vi "Calculate.vi"(5 "WFGraph Refnum":refnum<vi>, 7 "Measurement info":T2={"Det index"=0, "Clk index"=1, "Avg range"=1e-08}, 8 "error in":errorcluster, 9 "Changed reg":u8, 10 "Polarity":T1, 11 "file (use dialog)":path) -> (0 "error out":errorcluster, 2 "Settling time 5% (us)":dbl, 3 "Transition duration 10% (us)":dbl, 4 "Waveform data out":cluster{"t0":dbl, "dt":dbl, "Y":dbl[]}[](graph), 6 "Timing measurements":T3 {"measurement info 10%"."ref levels"."ref units" items=["absolute", "relative"]; "measurement info 5%"."ref levels"."ref units" items=["absolute", "relative"]})   [LabVIEW 2020]
uses:
  Timing measurements.ctl
  <vilib>/Waveform/WDTOps.llb/WDT Get Waveform Time Array DBL.vi
  <vilib>/measure/mascope.llb/Amplitude and Levels 1 chan.vi
  <vilib>/measure/mascope.llb/Transition Measurements 1 chan.vi
  <vilib>/Waveform/WDTOps.llb/WDT Waveform Duration DBL.vi
  <vilib>/Waveform/WDTOps.llb/WDT Get Waveform Subset DBL.vi
  <vilib>/Waveform/DWDTOps.llb/DWDT Analog to Digital.vi
  <vilib>/Waveform/DWDTOps.llb/DWDT Digital to Boolean Array.vi
  <vilib>/measure/NI_MAPro.lvlib
panel:
  out "full-scale range (pk-pk)":dbl=1.8
  out "# of clk edge":i32
  out "t0 to 10% (us)":dbl
  out "t0 to 5% (us)":dbl
  out "Settling index":i32
  out "measurement info 5%":T4 {"ref levels"."ref units" items=["absolute", "relative"]; "ref levels"."high ref level" format="%.2p"; "ref levels"."low ref level" format="%.2p"; "ref levels"."mid ref level" format="%.2p"; "end time" format="%.2p"; "start time" format="%.2p"}
  out "post-transition 5%":T5
  out "pre-transition 5%":T5
  out "slope 5%":dbl
  out "transition duration 5%":dbl
  out "amplitude":dbl format="%.2p"
  out "high state level":dbl format="%.2g"
  out "low state level":dbl format="%.2g"
  out "slope 10%":dbl
  out "measurement info 10%":T4 {"ref levels"."ref units" items=["absolute", "relative"]; "ref levels"."high ref level" format="%.2p"; "ref levels"."low ref level" format="%.2p"; "ref levels"."mid ref level" format="%.2p"; "end time" format="%.2p"; "start time" format="%.2p"}
  out "pre-transition 10%":T5
  out "Post-transition 10%":T5
  out "t0 (s)":dbl
  out "Digital Waveform Graph":digitalwaveform(graph)
  out "t0 index":i32
  # "Standard frame: 22nd\nExtended frame: 31st and 40th"
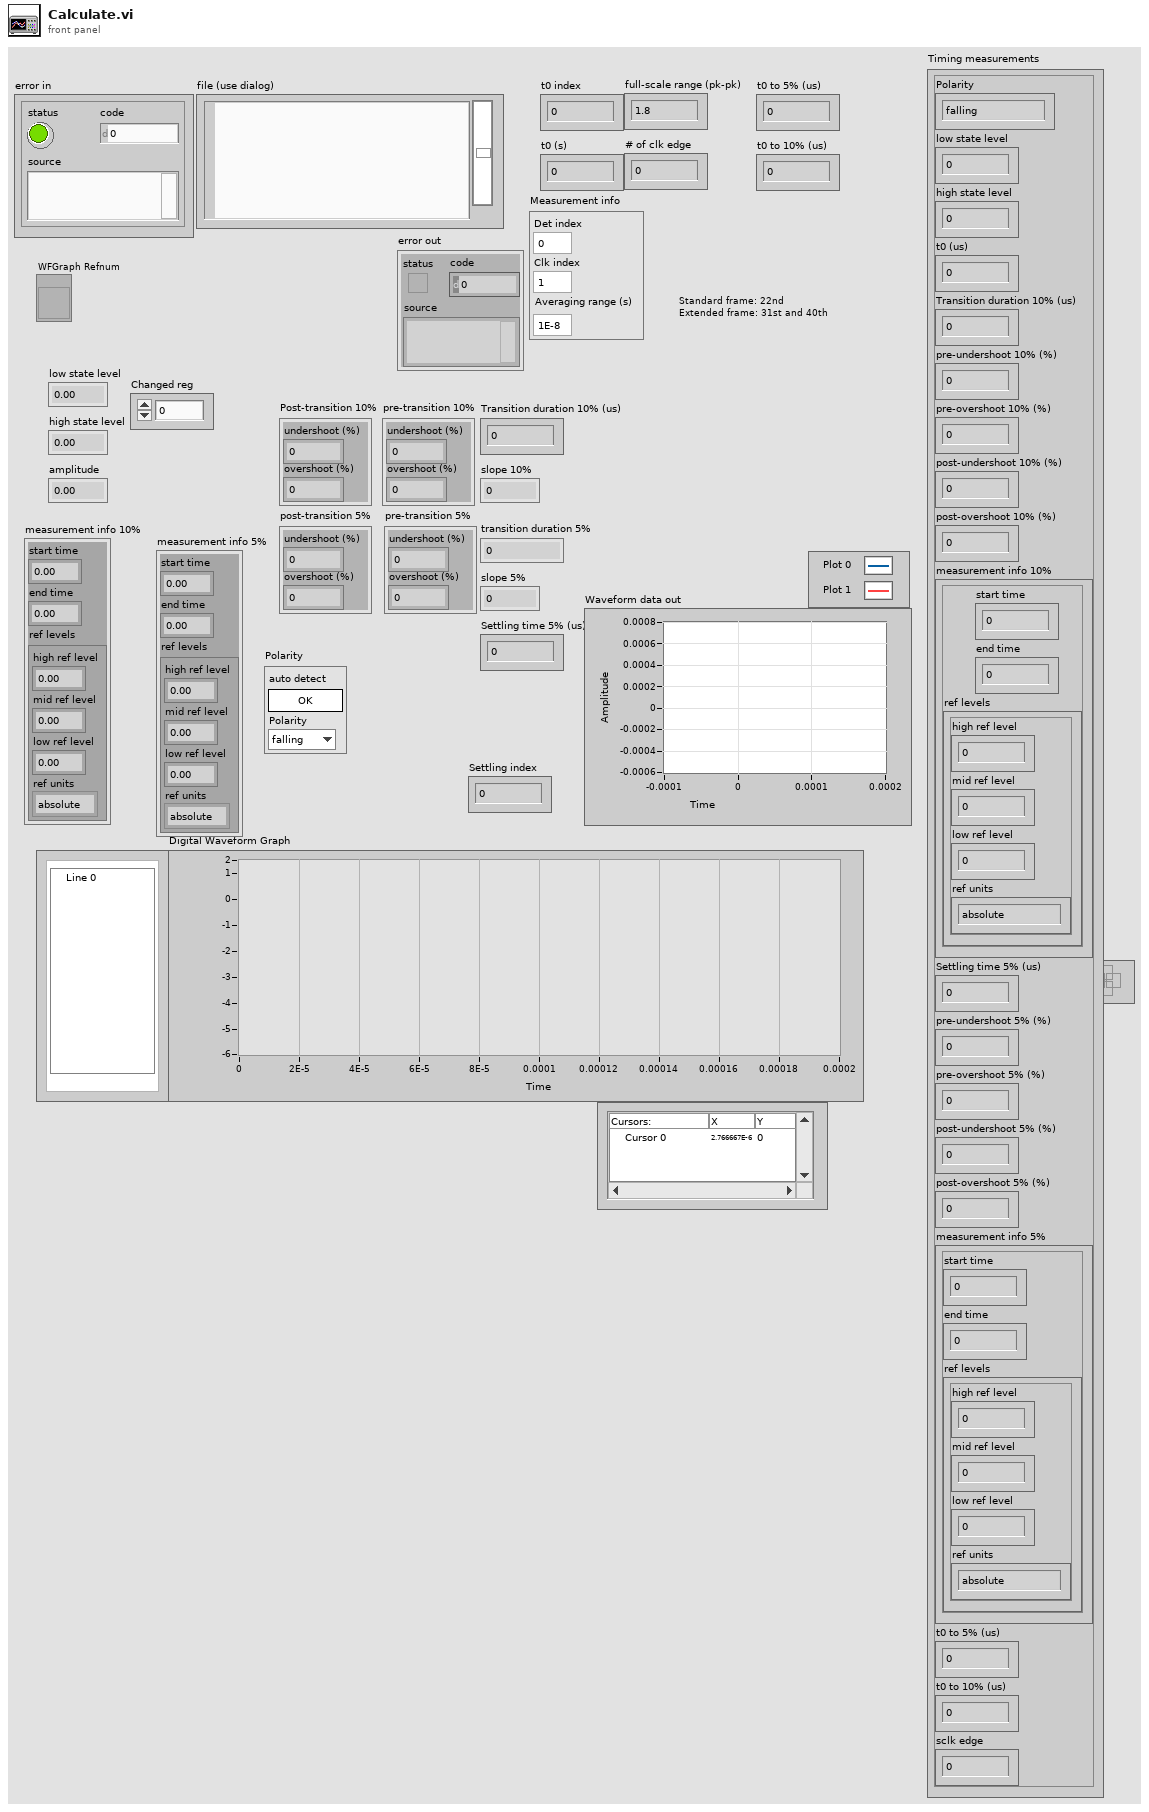
[diagram p1: front panel]
types:
  T1 = cluster{"auto detect":bool, "Polarity":enum16{"falling", "rising"}}
  T2 = cluster{"Det index":i32, "Clk index":i32, "Avg range":dbl}
  T3 = typedef "Timing measurements.ctl" = cluster{"Polarity":enum16{"falling", "rising"}, "low state level":dbl, "high state level":dbl, "t0 (us)":dbl, "Transition duration 10% (us)":dbl, "pre-undershoot 10% (%)":dbl, "pre-overshoot 10% (%)":dbl, "post-undershoot 10% (%)":dbl, "post-overshoot 10% (%)":dbl, "measurement info 10%":cluster{"start time":dbl, "end time":dbl, "ref levels":cluster{"high ref level":dbl, "mid ref level":dbl, "low ref level":dbl, "ref units":u16}}, "Settling time 5% (us)":dbl, "pre-undershoot 5% (%)":dbl, "pre-overshoot 5% (%)":dbl, "post-undershoot 5% (%)":dbl, "post-overshoot 5% (%)":dbl, "measurement info 5%":cluster{"start time":dbl, "end time":dbl, "ref levels":cluster{"high ref level":dbl, "mid ref level":dbl, "low ref level":dbl, "ref units":u16}}, "t0 to 5% (us)":dbl, "t0 to 10% (us)":dbl, "sclk edge":i32}
  T4 = cluster{"start time":dbl, "end time":dbl, "ref levels":cluster{"high ref level":dbl, "mid ref level":dbl, "low ref level":dbl, "ref units":u16}}
  T5 = cluster{"undershoot (%)":dbl, "overshoot (%)":dbl}
  T6 = cluster{"method":enum32{"histogram", "peak", "auto select"}, "histogram size":i32, "histogram method":enum16{"mode"}, "reserved":dbl}
  T7 = cluster{"high ref level":dbl, "mid ref level":dbl, "low ref level":dbl, "ref units":u16}
  T8 = typedef "imagedata.ctl" = cluster{"image type":i32, "image depth":i32, "image":u8[], "mask":u8[], "colors":u32[], "Rectangle":cluster{"left":i16, "top":i16, "right":i16, "bottom":i16}}
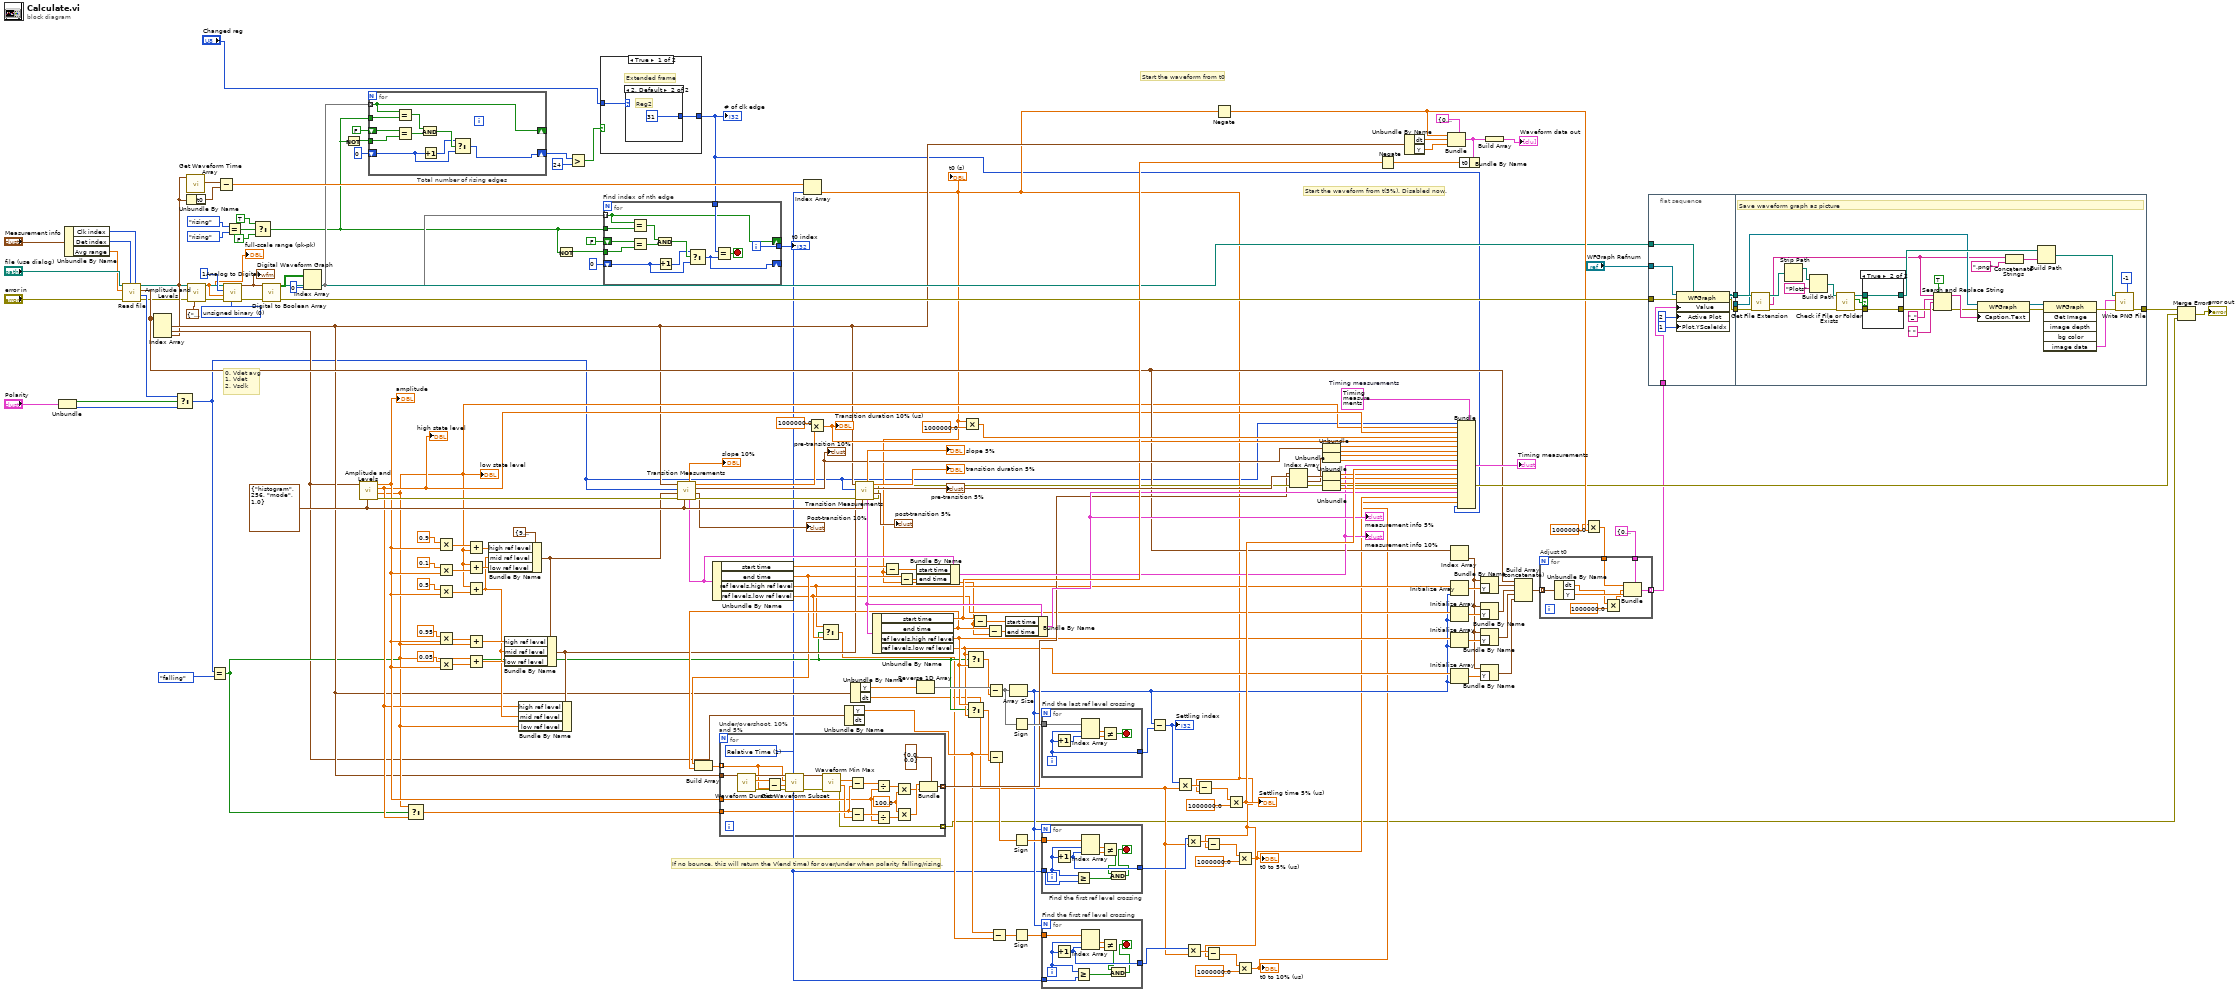
[diagram p0: block diagram]
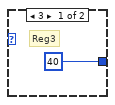
[diagram p2: hidden frame]
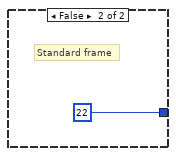
[diagram p3: hidden frame]
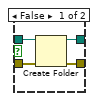
[diagram p4: hidden frame]
diagram:
  w117 = T3 {"Polarity"=enum."rising", "low state level"=0.0, "high state level"=0.0, "t0 (us)"=0.0, "Transition duration 10% (us)"=0.0, "pre-undershoot 10% (%)"=0.0, "pre-overshoot 10% (%)"=0.0, "post-undershoot 10% (%)"=0.0, "post-overshoot 10% (%)"=0.0, "measurement info 10%"={"start time"=0.0, "end time"=0.0, "ref levels"={"high ref level"=0.0, "mid ref level"=0.0, "low ref level"=0.0, "ref units"=0}}, "Settling time 5% (us)"=0.0, "pre-undershoot 5% (%)"=0.0, "pre-overshoot 5% (%)"=0.0, "post-undershoot 5% (%)"=0.0, "post-overshoot 5% (%)"=0.0, "measurement info 5%"={"start time"=0.0, "end time"=0.0, "ref levels"={"high ref level"=0.0, "mid ref level"=0.0, "low ref level"=0.0, "ref units"=0}}, "t0 to 5% (us)"=0.0, "t0 to 10% (us)"=0.0, "sclk edge"=0}  # Timing measurements
  w140 = T6 {"method"=enum."histogram", "histogram size"=256, "histogram method"=enum."mode", "reserved"=1.0} ("state settings")
  w177 = u16 0 items=["unsigned binary", "offset binary", "2's complement"] ("data format (offset binary)")
  # "If no bounce, this will return the V(end time) for over/under when polarity falling/rising."
  # "0. Vdet avg\n1. Vdet\n2. Vsclk"
  # "Start the waveform from t(5%). Disabled now."
  # "Start the waveform from t0"
  n1 = Unbundle("Polarity") -> ("auto detect"=w21:bool, "Polarity"=w20:enum16{"falling", "rising"})
  n2 = Unbundle By Name("Measurement info") -> ("Clk index"=w28:i32, "Det index"=w27:i32, "Avg range"=w2:dbl)
  n3 = call "Read file.vi"("Clk index"=w28, "Det index"=w27, "error in (no error)"="error in", "Averaging range"=w2, "file (use dialog) in"="file (use dialog)") -> ("Error Out"=w3:errorcluster, "Polarity"=w19:enum16{"falling", "rising"}, "Waveform Array"=w68:waveform(dbl)[], "file (use dialog) out"=w69:path)  [unwired: 3 in]
  n4 = Index Array(array=w68) -> (element #1=w58:waveform(dbl), element #2=w33:waveform(dbl), element #3=w7:waveform(dbl))  [unwired: 3 in]
  n5 = Select(t=w19, s=w21, f=w20) -> (s? t:f=w18:enum16{"falling", "rising"})
  n6 = call-poly <vilib>:"Get Waveform Time Array.vi"("waveform in"=w7) -> ("X array"=w170:timestamp[])  [unwired: 9 in, 1 out]
  n7 = Unbundle By Name(w7) -> ("t0"=w171:timestamp)
  n8 = call-poly <vilib>:"Amplitude and Levels.vi"("state settings"=T6 {"method"=enum."histogram", "histogram size"=256, "histogram method"=enum."mode", "reserved"=1.0}, "error in (no error)"=w3, "signal in"=w7) -> ("error out"=w6:errorcluster, "amplitude"=w4:dbl)  [unwired: 5 in, 2 out]
  "full-scale range (pk-pk)" <- w4
  n9 = Equal?(x=w18, y=enum16{"falling", "rising"}."falling" ("Polarity 2")) -> (x = y?=w45:bool)
  n10 = Subtract(x=w170, y=w171) -> (x-y=w169:dbl[])
  n11 = call-poly <vilib>:"Analog to Digital.vi"("data format (offset binary)"=w177, "error in (no error)"=w6, "full-scale range (pk-pk)"=w4, "resolution (16 bit)"=1, "analog waveform"=w7) -> ("error out"=w176:errorcluster, "digital waveform"=w152:digitalwaveform)  [unwired: 3 in, 2 out]
  "Digital Waveform Graph" <- w152
  n12 = Equal?(x=enum16{"falling", "rising"}."rising" ("clk edge"), y=enum16{"falling", "rising"}."rising") -> (x = y?=w136:bool)
  n13 = Select(t=TRUE ("x"), s=w136, f=FALSE ("y")) -> (s? t:f=w12:bool)
  n14 = call-poly <vilib>:"Digital to Boolean Array.vi"("error in (no error)"=w176, "digital waveform"=w152) -> ("error out"=w159:errorcluster, "boolean array"=w173:bool[][])  [unwired: 8 in]
  n15 = Index Array(array=w173, index (col)=0 ("disabled index (col)")) -> (element=w14:bool[])  [unwired: 1 in]
  n16 = Not(x=w12) -> (.not. x?=w13:bool)
  n17 = call-poly <vilib>:"Amplitude and Levels.vi"("state settings"=w140, "signal in"=w33) -> ("error out"=w162:errorcluster, "low state level"=w63:dbl, "high state level"=w65:dbl, "amplitude"=w78:dbl)  [unwired: 6 in]
  "low state level" <- w63
  "high state level" <- w65
  "amplitude" <- w78
  n18 = for "Total number of rising edges" {
    shift-right: [w181] -> _
    shift-left: FALSE ("Boolean") -> [w182]
    tunnel: w14 -> [w181] mode=indexing
    shift-right: [w184] -> w9
    shift-left: 0 -> [w185]
    tunnel: w12 -> [w180]
    tunnel: w13 -> [w179]
    n19 = Equal?(x=w181, y=w180) -> (x = y?=w188:bool)
    n20 = Equal?(x=w182, y=w179) -> (x = y?=w183:bool)
    n21 = And(x=w188, y=w183) -> (x .and. y?=w187:bool)
    n22 = Increment(x=w185) -> (x+1=w186:i32)
    n23 = Select(t=w186, s=w187, f=w185) -> (s? t:f=w184:i32)
  }
  n24 = Select(t=w63, s=w45, f=w65) -> (s? t:f=w79:dbl)
  n25 = Multiply(x=0.9, y=w78) -> (x*y=w93:dbl)
  n26 = Multiply(x=0.1, y=w78) -> (x*y=w94:dbl)
  n27 = Multiply(x=0.5, y=w78) -> (x*y=w85:dbl)
  n28 = Multiply(x=0.95, y=w78) -> (x*y=w92:dbl)
  n29 = Multiply(x=0.05, y=w78) -> (x*y=w91:dbl)
  n30 = Add(x=w93, y=w63) -> (x+y=w87:dbl)
  n31 = Add(x=w63, y=w94) -> (x+y=w88:dbl)
  n32 = Add(x=w63, y=w85) -> (x+y=w66:dbl)
  n33 = Add(x=w92, y=w63) -> (x+y=w89:dbl)
  n34 = Add(x=w63, y=w91) -> (x+y=w90:dbl)
  n35 = Bundle By Name(cluster=T7 {"high ref level"=90.0, "mid ref level"=50.0, "low ref level"=10.0, "ref units"=0} ("reference levels"), "high ref level"=w87, "mid ref level"=w66, "low ref level"=w88) -> (w84:T7)
  n36 = Bundle By Name(cluster=w84, "high ref level"=w89, "mid ref level"=w66, "low ref level"=w90) -> (w64:T7)
  n37 = Bundle By Name(cluster=w64, "high ref level"=w65, "mid ref level"=w66, "low ref level"=w63) -> ()  [unwired: 1 out]
  n38 = Not(x=w12) -> (.not. x?=w135:bool)
  n39 = Greater?(x=w9, y=24) -> (0:w10:bool)
  n40 = case shown="True" w10 {
    tunnel: [w190 22 ("# of clk edge")] -> w8
    tunnel: "Changed reg" -> [w189 _]
    frame True {
      # "Extended frame"
      n41 = case shown="2, Default" w189 {
        tunnel: [40 ("# of clk edge") 31 ("# of clk edge")] -> w190
        frame 3 {
          # "Reg3"
        }
        frame 2, Default {
          # "Reg2"
        }
      }
    }
    frame False {
      # "Standard frame"
    }
  }
  "# of clk edge" <- w8
  n42 = for "Find index of nth edge" {
    shift-right: [w197] -> _
    shift-left: FALSE ("Boolean") -> [w198]
    tunnel: w14 -> [w197] mode=indexing
    shift-right: [w201] -> _
    shift-left: 0 -> [w203]
    tunnel: w8 -> [w200]
    tunnel: [w196] -> w30
    tunnel: w12 -> [w195]
    tunnel: w135 -> [w194]
    i -> [w196]
    stop <- w202 stop-if-true
    n43 = Equal?(x=w197, y=w195) -> (x = y?=w206:bool)
    n44 = Equal?(x=w198, y=w194) -> (x = y?=w199:bool)
    n45 = And(x=w206, y=w199) -> (x .and. y?=w205:bool)
    n46 = Increment(x=w203) -> (x+1=w204:i32)
    n47 = Select(t=w204, s=w205, f=w203) -> (s? t:f=w201:i32)
    n48 = Equal?(x=w200, y=w201) -> (x = y?=w202:bool)
  }
  "t0 index" <- w30
  n49 = call-poly <vilib>:"Transition Measurements.vi"("percent level settings"=w140, "error in (no error)"=w162, "reference levels"=w84, "polarity (rising)"=w18, "signal in"=w58) -> ("error out"=w100:errorcluster, "post-transition"=→"Post-transition 10%":T5, "pre-transition"=w124:T5, "transition duration"=w163:dbl, "measurement info"=w110:T4, "slope"=→"slope 10%":dbl)  [unwired: 1 in]
  "pre-transition 10%" <- w124
  n50 = Unbundle By Name(w110) -> ("start time"=w80:dbl, "end time"=w62:dbl, "ref levels.high ref level"=w46:dbl, "ref levels.low ref level"=w47:dbl)
  n51 = Index Array(array=w169, index=w30) -> (element=w34:dbl)
  "t0 (s)" <- w34
  n52 = Multiply(x=1000000.0 ("y"), y=w163) -> (x*y=w101:dbl)
  "Transition duration 10% (us)" <- w101
  n53 = Select(t=w46, s=w45, f=w47) -> (s? t:f=w43:dbl)
  n54 = Unbundle By Name(w33) -> ("Y"=w44:dbl[])  [unwired: 1 out]
  n55 = Unbundle By Name(w58) -> ("Y"=w48:dbl[], "dt"=w35:dbl)
  n56 = call-poly <vilib>:"Transition Measurements.vi"("percent level settings"=w140, "error in (no error)"=w100, "reference levels"=w64, "polarity (rising)"=w18, "signal in"=w58) -> ("error out"=w81:errorcluster, "post-transition"=→"post-transition 5%":T5, "pre-transition"=w123:T5, "transition duration"=→"transition duration 5%":dbl, "measurement info"=w105:T4, "slope"=→"slope 5%":dbl)  [unwired: 1 in]
  "pre-transition 5%" <- w123
  n57 = Unbundle By Name(w105) -> ("start time"=w104:dbl, "end time"=w77:dbl, "ref levels.high ref level"=w57:dbl, "ref levels.low ref level"=w56:dbl)
  n58 = Build Array(w62, w77) -> (w76:dbl[])
  n59 = for "Under/overshoot, 10% and 5%" {
    tunnel: w58 -> [w227]
    tunnel: w79 -> [w218]
    tunnel: w78 -> [w215]
    tunnel: w76 -> [w208] mode=indexing
    tunnel: [w212] -> w75 mode=indexing
    tunnel: [w210] -> w23 mode=indexing
    w216 = 100.0 ("y")
    w229 = u16 1 items=["Samples", "Relative Time"] ("start/duration format")
    n60 = call-poly <vilib>:"Waveform Duration.vi"("waveform in"=w227) -> ("error out"=w225:errorcluster, "duration"=w209:dbl, "waveform out"=w226:waveform(dbl))  [unwired: 8 in]
    n61 = Subtract(x=w209, y=w208) -> (x-y=w207:dbl)
    n62 = call-poly <vilib>:"Get Waveform Subset.vi"("start/duration format"=w229, "error in (no error)"=w225, "duration"=w207, "start samples/time"=w208, "waveform in"=w226) -> ("error out"=w228:errorcluster, "waveform out"=w224:waveform(dbl))  [unwired: 1 in, 2 out]
    n63 = call <vilib>:"Waveform Min Max.vi"("error in (no error)"=w228, "waveform in"=w224) -> ("error out"=w210:errorcluster, "Y min"=w217:dbl, "Y max"=w223:dbl)  [unwired: 4 in, 3 out]
    n64 = Subtract(x=w223, y=w218) -> (x-y=w219:dbl)
    n65 = Subtract(x=w218, y=w217) -> (x-y=w220:dbl)
    n66 = Divide(x=w219, y=w215) -> (x/y=w222:dbl)
    n67 = Divide(x=w220, y=w215) -> (x/y=w221:dbl)
    n68 = Multiply(x=w222, y=w216) -> (x*y=w213:dbl)
    n69 = Multiply(x=w216, y=w221) -> (x*y=w214:dbl)
    n70 = Bundle(cluster=T5 {"undershoot (%)"=0.0, "overshoot (%)"=0.0} ("post-transition"), "undershoot (%)"=w214, "overshoot (%)"=w213) -> (w212:T5)
  }
  n71 = Subtract(x=w80, y=w34) -> (x-y=w109:dbl)
  n72 = Subtract(x=w62, y=w34) -> (x-y=w108:dbl)
  n73 = Reverse 1D Array(array=w48) -> (reversed array=w158:dbl[])
  n74 = Bundle By Name(cluster=w110, "start time"=w109, "end time"=w108) -> (w102:T4)
  "measurement info 10%" <- w102
  n75 = Multiply(x=w34, y=1000000.0) -> (x*y=w114:dbl)
  n76 = Select(t=w56, s=w45, f=w57) -> (s? t:f=w157:dbl)
  n77 = Select(t=w57, s=w45, f=w56) -> (s? t:f=w55:dbl)
  n78 = Subtract(x=w104, y=w34) -> (x-y=w106:dbl)
  n79 = Subtract(x=w77, y=w34) -> (x-y=w107:dbl)
  n80 = Subtract(x=w158, y=w157) -> (x-y=w155:dbl[])
  n81 = Subtract(x=w44, y=w55) -> (x-y=w53:dbl[])
  n82 = Subtract(x=w44, y=w43) -> (x-y=w40:dbl[])
  n83 = Bundle By Name(cluster=w105, "start time"=w106, "end time"=w107) -> (w103:T4)
  "measurement info 5%" <- w103
  n84 = Array Size(array=w155) -> (size(s)=w41:i32)
  n85 = Sign(1:w155) -> (0:w156:dbl[])
  n86 = Sign(1:w53) -> (0:w54:dbl[])
  n87 = Sign(1:w40) -> (0:w42:dbl[])
  n88 = for "Find the last ref level crossing" {
    N: w41 -> [_]
    tunnel: w156 -> [w235]
    tunnel: [w230] -> w154
    i -> [w230]
    stop <- w231 stop-if-true
    n89 = Increment(x=w230) -> (x+1=w234:i32)
    n90 = Index Array(array=w235, index #1=w230, index #2=w234) -> (element #1=w233:dbl, element #2=w232:dbl)
    n91 = Not Equal?(x=w233, y=w232) -> (x != y?=w231:bool)
  }
  n92 = for "Find the first ref level crossing" {
    N: w41 -> [_]
    tunnel: w54 -> [w244]
    tunnel: [w241] -> w49
    tunnel: w30 -> [w238]
    i -> [w239]
    stop <- w236 stop-if-true
    n93 = Increment(x=w239) -> (x+1=w241:i32)
    n94 = Greater Or Equal?(x=w239, y=w238) -> (x >= y?=w237:bool)
    n95 = Index Array(array=w244, index #1=w239, index #2=w241) -> (element #1=w243:dbl, element #2=w242:dbl)
    n96 = Not Equal?(x=w243, y=w242) -> (x != y?=w240:bool)
    n97 = And(x=w240, y=w237) -> (x .and. y?=w236:bool)
  }
  n98 = for "Find the first ref level crossing" {
    N: w41 -> [_]
    tunnel: w42 -> [w253]
    tunnel: [w250] -> w36
    tunnel: w30 -> [w248]
    i -> [w247]
    stop <- w246 stop-if-true
    n99 = Increment(x=w247) -> (x+1=w250:i32)
    n100 = Greater Or Equal?(x=w247, y=w248) -> (x >= y?=w249:bool)
    n101 = Index Array(array=w253, index #1=w247, index #2=w250) -> (element #1=w252:dbl, element #2=w251:dbl)
    n102 = Not Equal?(x=w252, y=w251) -> (x != y?=w245:bool)
    n103 = And(x=w245, y=w249) -> (x .and. y?=w246:bool)
  }
  n104 = Subtract(x=w41, y=w154) -> (x-y=w153:i32)
  "Settling index" <- w153
  n105 = Multiply(x=w153, y=w35) -> (x*y=w142:dbl)
  n106 = Multiply(x=w49, y=w35) -> (x*y=w51:dbl)
  n107 = Multiply(x=w36, y=w35) -> (x*y=w38:dbl)
  n108 = Subtract(x=w142, y=w34) -> (x-y=w141:dbl)
  n109 = Subtract(x=w51, y=w34) -> (x-y=w52:dbl)
  n110 = Subtract(x=w38, y=w34) -> (x-y=w37:dbl)
  n111 = Negate(x=w34) -> (-x=w83:dbl)
  n112 = Multiply(x=w141, y=1000000.0) -> (x*y=w125:dbl)
  "Settling time 5% (us)" <- w125
  n113 = Multiply(x=w52, y=1000000.0) -> (x*y=w32:dbl)
  "t0 to 5% (us)" <- w32
  n114 = Multiply(x=w37, y=1000000.0) -> (x*y=w31:dbl)
  "t0 to 10% (us)" <- w31
  n115 = Index Array(array=w75) -> (element #1=w74:T5, element #2=w73:T5)  [unwired: 2 in]
  n116 = Unbundle(w124) -> ("undershoot (%)"=w129:dbl, "overshoot (%)"=w128:dbl)
  n117 = Unbundle(w74) -> ("undershoot (%)"=w127:dbl, "overshoot (%)"=w126:dbl)
  n118 = Unbundle(w123) -> ("undershoot (%)"=w121:dbl, "overshoot (%)"=w120:dbl)
  n119 = Unbundle(w73) -> ("undershoot (%)"=w119:dbl, "overshoot (%)"=w118:dbl)
  n120 = Negate(x=w104) -> (-x=w113:dbl)
  n121 = Unbundle By Name(w58) -> ("dt"=w131:dbl, "Y"=w130:dbl[])
  n122 = Bundle(cluster=cluster{"t0":dbl, "dt":dbl, "Y":dbl[]} {"t0"=0.0, "dt"=0.0, "Y"=[]}, "t0"=w83, "dt"=w131, "Y"=w130) -> (w112:cluster{"t0":dbl, "dt":dbl, "Y":dbl[]})
  n123 = Index Array(array=w68) -> (element=w147:waveform(dbl))  [unwired: 1 in]
  n124 = Initialize Array(w46, w41) -> (w151:dbl[])
  n125 = Initialize Array(w47, w41) -> (w148:dbl[])
  n126 = Initialize Array(w57, w41) -> (w149:dbl[])
  n127 = Initialize Array(w56, w41) -> (w150:dbl[])
  n128 = Bundle(cluster=w117, "Polarity"=w18, "low state level"=w63, "high state level"=w65, "t0 (us)"=w114, "Transition duration 10% (us)"=w101, "pre-undershoot 10% (%)"=w129, "pre-overshoot 10% (%)"=w128, "post-undershoot 10% (%)"=w127, "post-overshoot 10% (%)"=w126, "measurement info 10%"=w102, "Settling time 5% (us)"=w125, "pre-undershoot 5% (%)"=w121, "pre-overshoot 5% (%)"=w120, "post-undershoot 5% (%)"=w119, "post-overshoot 5% (%)"=w118, "measurement info 5%"=w103, "t0 to 5% (us)"=w32, "t0 to 10% (us)"=w31, "sclk edge"=w8) -> (→"Timing measurements":T3)
  n129 = Bundle By Name(cluster=w112, "t0"=w113) -> ()  [unwired: 1 out]
  n130 = Bundle By Name(cluster=w147, "Y"=w151) -> (w146:waveform(dbl))
  n131 = Bundle By Name(cluster=w147, "Y"=w148) -> (w145:waveform(dbl))
  n132 = Bundle By Name(cluster=w147, "Y"=w149) -> (w144:waveform(dbl))
  n133 = Bundle By Name(cluster=w147, "Y"=w150) -> (w143:waveform(dbl))
  n134 = Build Array(w112) -> (→"Waveform data out":cluster{"t0":dbl, "dt":dbl, "Y":dbl[]}[])
  n135 = Build Array (concatenate)(w68, w146, w145, w144, w143) -> (w61:waveform(dbl)[])
  n136 = Multiply(x=1000000.0 ("y"), y=w83) -> (x*y=w59:dbl)
  n137 = for "Adjust t0" {
    tunnel: w61 -> [w258] mode=indexing
    tunnel: cluster{"t0":dbl, "dt":dbl, "Y":dbl[]} {"t0"=0.0, "dt"=0.0, "Y"=[]} -> [w261]
    tunnel: [w259] -> w24 mode=indexing
    tunnel: w59 -> [w254]
    n138 = Unbundle By Name(w258) -> ("dt"=w256:dbl, "Y"=w260:dbl[])
    n139 = Multiply(x=w256, y=1000000.0) -> (x*y=w255:dbl)
    n140 = Bundle(cluster=w261, "t0"=w254, "dt"=w255, "Y"=w260) -> (w259:cluster{"t0":dbl, "dt":dbl, "Y":dbl[]})
  }
  n141 = flat-sequence {
    tunnel: w24 -> [w262]
    tunnel: w159 -> [w265]
    tunnel: w69 -> [w269]
    tunnel: [w269] -> w134
    tunnel: [w264] -> w133
    tunnel: "WFGraph Refnum" -> [w268]
    tunnel: [w263] -> w25
    tunnel: [w279] -> w161
    tunnel: w134 -> [w297]
    tunnel: w133 -> [w284]
    tunnel: w25 -> [w280]
    frame #0 {
      n142 = property class="WFGraph"(reference=w268, error in=w265, "Value"=w262, "Active Plot"=u32 2, "Plot.YScaleIdx"=u32 1 ("Plot.Y Scale Index")) -> (reference out=w263:refnum<vi>, error out=w264:errorcluster)
    }
    frame #1 {
      # "Save waveform graph as picture"
      n143 = call <vilib>:"Get File Extension.vi"("error in (no error)"=w284, "file"=w297) -> ("error out"=w292:errorcluster, "filename without extension"=w272:string, "dup file"=w296:path)  [unwired: 5 in, 2 out]
      n144 = Strip Path(path=w296) -> (stripped path=w286:path)  [unwired: 1 out]
      n145 = Build Path(base path=w286, name or relative path="Plots") -> (appended path=w291:path)
      n146 = call <vilib>:"Check if File or Folder Exists.vi"("error in (no error)"=w292, "path"=w291) -> ("error out"=w289:errorcluster, "file or folder exists?"=w290:bool, "dup path"=w288:path)  [unwired: 7 in]
      n147 = case shown="True" w290 {
        tunnel: w289 -> [w301 w303]
        tunnel: w288 -> [w300 w302]
        tunnel: [w299 w303] -> w287
        tunnel: [w298 w302] -> w285
        frame False {
          n148 = Create Folder(path (use dialog)=w300, error in=w301) -> (created path=w298:path, error out=w299:errorcluster)  [unwired: 1 in, 1 out]
        }
        frame True {
        }
      }
      n149 = Search and Replace String(replace all?=TRUE ("replace all? (F)"), input string=w272, search string="_", replace string=" " ("replace string (\"\")"), error in=w287) -> (result string=w282:string, error out=w281:errorcluster)  [unwired: 3 in, 2 out]
      n150 = property class="WFGraph"(reference=w280, error in=w281, "Caption.Text"=w282) -> (reference out=w276:refnum<vi>, error out=w275:errorcluster)
      n151 = Concatenate Strings(w272, ".png" ("string")) -> (w271:string)
      n152 = Build Path(base path=w285, name or relative path=w271) -> (appended path=w278:path)
      n153 = invoke class="WFGraph" method="Get Image"(reference=w276, error in=w275) -> (error out=w274:errorcluster, "image data"=w273:T8)  [unwired: 4 in, 4 out]
      n154 = call <vilib>:"Write PNG File.vi"("compression (default)"=-1, "error in (no error)"=w274, "image data"=w273, "path to PNG file"=w278) -> ("error out"=w279:errorcluster)  [unwired: 6 in, 1 out]
    }
  }
  n155 = Merge Errors(w161, w81, w23) -> (→"error out":errorcluster)
